vi "Decode.vi"(2 "Data":dbl[](array[numeric]), 8 "error in (no error)":errorcluster, 10 "Message in":string, 11 "Ultrasonic Sensor in":refnum<class "Ultrasonic Sensor.lvclass">) -> (0 "error out":errorcluster, 3 "Ultrasonic Sensor out":refnum<class "Ultrasonic Sensor.lvclass">)   [LabVIEW 2021, in "Ultrasonic Sensor.lvclass"]
uses:
  Ultrasonic Sensor.lvclass
  Sensor/Sensor.lvclass
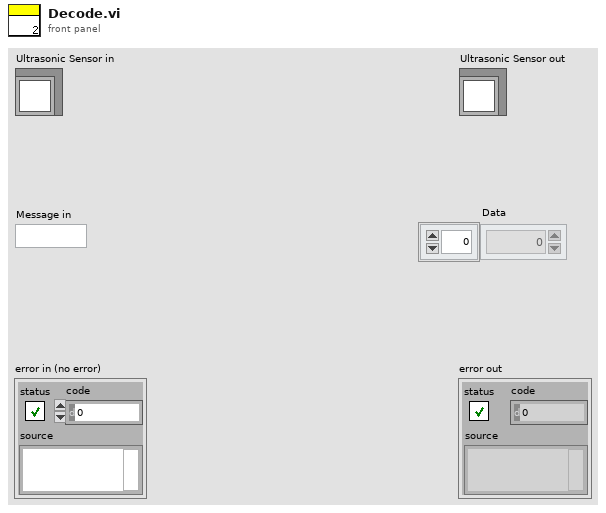
[diagram p1: front panel]
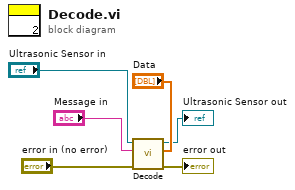
[diagram p0: block diagram]
diagram:
  n1 = call-parent "Decode.vi"("Data"="Data", "error in (no error)"="error in (no error)", "Message in"="Message in", "Sensor in"="Ultrasonic Sensor in") -> ("error out"=→"error out":errorcluster, "Sensor out"=→"Ultrasonic Sensor out":refnum<class "Ultrasonic Sensor.lvclass">)  [unwired: 6 in]
